vi "lapdata.vi"(6 "Reset":bool, 7 "Laptrigger":bool, 8 "InverterTemps":dbl[](array[numeric]), 9 "MotorTemps":dbl[](array[numeric]), 10 "Current":dbl, 11 "SoC":i32) -> (0 "Inverter Temp":cluster{i32[], dbl[]}[](graph), 1 "Motor Temp":cluster{i32[], dbl[]}[](graph), 3 "Lap                    Laptime                        SoC                 Current Avg |                             Motor Temperatures                          |                               Inverter Temperatures":T1(array[cluster]) {"Laptime" format="%<%M:%S%2u>T"})   [LabVIEW 2017]
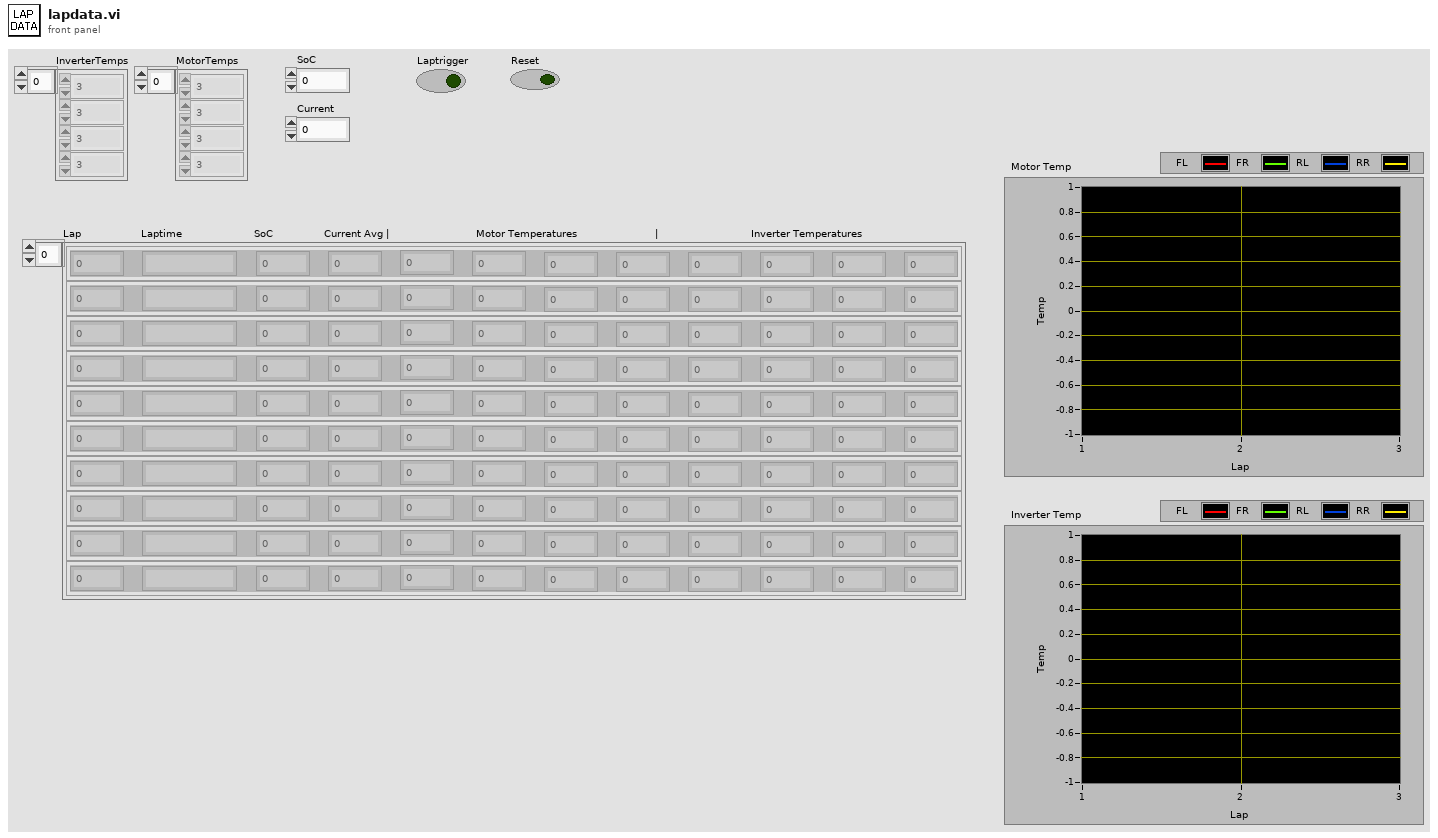
[diagram p1: front panel]
types:
  T1 = cluster{"SoC":i32, "MotorTemp_FL":dbl, "MotorTemp_FR":dbl, "MotorTemp_RL":dbl, "MotorTemp_RR":dbl, "InverterTemp_FL":dbl, "InverterTemp_FR":dbl, "InverterTemp_RL":dbl, "InverterTemp_RR":dbl, "Laptime":timestamp, "Lap":i32, "Curr Abs Avg":dbl}[]
  T2 = cluster{"SoC":i32, "MotorTemp_FL":dbl, "MotorTemp_FR":dbl, "MotorTemp_RL":dbl, "MotorTemp_RR":dbl, "InverterTemp_FL":dbl, "InverterTemp_FR":dbl, "InverterTemp_RL":dbl, "InverterTemp_RR":dbl, "Laptime":timestamp, "Lap":i32, "Current Abs Avg":dbl}[]
  T3 = cluster{"SoC":i32, "MotorTemp_FL":dbl, "MotorTemp_FR":dbl, "MotorTemp_RL":dbl, "MotorTemp_RR":dbl, "InverterTemp_FL":dbl, "InverterTemp_FR":dbl, "InverterTemp_RL":dbl, "InverterTemp_RR":dbl, "Laptime":timestamp, "Lap":i32, "Current Abs Avg":dbl}
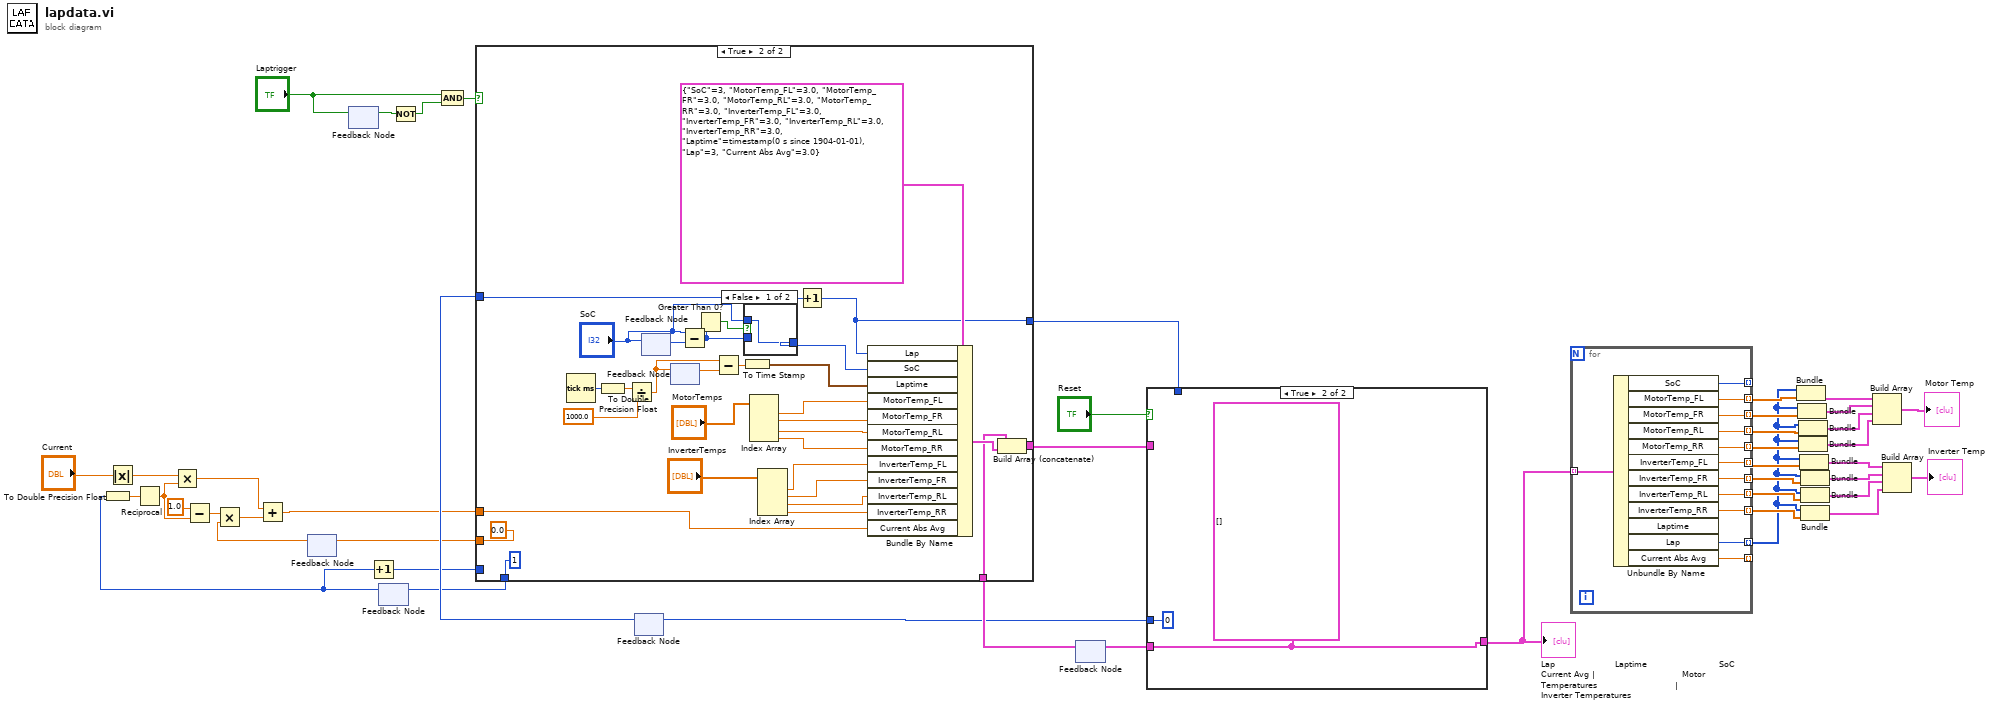
[diagram p0: block diagram]
diagram:
  n1 = Absolute Value(x="Current") -> (abs(x)=w26:dbl)
  n2 = feedback #1() -> (w30:dbl)  [unwired: 1 in]
  n3 = feedback #2() -> (w44:bool)  [unwired: 1 in]
  n4 = feedback-in #2("Laptrigger") -> ()
  n5 = feedback #3() -> (w33:i32)  [unwired: 1 in]
  n6 = To Double Precision Float(number=w33) -> (double precision float=w34:dbl)
  n7 = Reciprocal(x=w34) -> (1/x=w28:dbl)
  n8 = Multiply(x=w26, y=w28) -> (x*y=w32:dbl)
  n9 = Subtract(x=1.0, y=w28) -> (x-y=w29:dbl)
  n10 = Multiply(x=w29, y=w30) -> (x*y=w31:dbl)
  n11 = Add(x=w32, y=w31) -> (x+y=w22:dbl)
  n12 = Increment(x=w33) -> (x+1=w24:i32)
  n13 = Not(x=w44) -> (.not. x?=w43:bool)
  n14 = And(x="Laptrigger", y=w43) -> (x .and. y?=w41:bool)
  n15 = feedback #4() -> (w35:i32)  [unwired: 1 in]
  n16 = feedback #5() -> (w45:T2)  [unwired: 1 in]
  n17 = case shown="True" w41 {
    tunnel: w45 -> [w49 w60]
    tunnel: [w49 w79] -> w39
    tunnel: [w48 w58] -> w37
    tunnel: w35 -> [w48 w59]
    tunnel: w24 -> [w47 _]
    tunnel: [w47 1 ("Lap")] -> w23
    tunnel: w22 -> [w46 w54]
    tunnel: [w46 0.0] -> w21
    frame False {
    }
    frame True {
      n18 = Tick Count (ms)() -> (millisecond timer value=w68:u32)
      n19 = To Double Precision Float(number=w68) -> (double precision float=w67:dbl)
      n20 = Divide(x=w67, y=1000.0) -> (x/y=w64:dbl)
      n21 = feedback #6() -> (w57:i32)  [unwired: 1 in]
      n22 = feedback-in #6("SoC") -> ()
      n23 = feedback #7() -> (w65:dbl)  [unwired: 1 in]
      n24 = feedback-in #7(w64) -> ()
      n25 = Subtract(x="SoC", y=w57) -> (x-y=w52:i32)
      n26 = Greater Than 0?(x=w52) -> (x > 0?=w51:bool)
      n27 = Subtract(x=w64, y=w65) -> (x-y=w63:dbl)
      n28 = To Time Stamp(1:w63) -> (0:w62:timestamp)
      n29 = case shown="False" w51 {
        tunnel: w52 -> [_ w82]
        tunnel: [w81 w82] -> w53
        tunnel: "SoC" -> [w81 _]
        frame False {
        }
        frame True {
        }
      }
      n30 = Index Array(array="MotorTemps") -> (element #1=w77:dbl, element #2=w76:dbl, element #3=w75:dbl, element #4=w74:dbl)  [unwired: 4 in]
      n31 = Index Array(array="InverterTemps") -> (element #1=w72:dbl, element #2=w71:dbl, element #3=w70:dbl, element #4=w69:dbl)  [unwired: 4 in]
      n32 = Increment(x=w59) -> (x+1=w58:i32)
      n33 = Bundle By Name(cluster=T3 {"SoC"=3, "MotorTemp_FL"=3.0, "MotorTemp_FR"=3.0, "MotorTemp_RL"=3.0, "MotorTemp_RR"=3.0, "InverterTemp_FL"=3.0, "InverterTemp_FR"=3.0, "InverterTemp_RL"=3.0, "InverterTemp_RR"=3.0, "Laptime"=timestamp(0 s since 1904-01-01), "Lap"=3, "Current Abs Avg"=3.0}, "Lap"=w58, "SoC"=w53, "Laptime"=w62, "MotorTemp_FL"=w77, "MotorTemp_FR"=w76, "MotorTemp_RL"=w75, "MotorTemp_RR"=w74, "InverterTemp_FL"=w72, "InverterTemp_FR"=w71, "InverterTemp_RL"=w70, "InverterTemp_RR"=w69, "Current Abs Avg"=w54) -> (w61:T3)
      n34 = Build Array (concatenate)(w60, w61) -> (w79:T2)
    }
  }
  n35 = feedback-in #1(w21) -> ()
  n36 = feedback-in #3(w23) -> ()
  n37 = case shown="True" "Reset" {
    tunnel: [w84 w85] -> w38
    tunnel: w39 -> [w84 _]
    tunnel: [w84 w85] -> w20
    tunnel: w37 -> [w83 _]
    tunnel: [w83 0 ("Lap")] -> w36
    frame False {
    }
    frame True {
      w85 = T2 []
    }
  }
  "Lap                    Laptime                        SoC                 Current Avg |                             Motor Temperatures                          |                               Inverter Temperatures" <- w20
  n38 = feedback-in #4(w36) -> ()
  n39 = feedback-in #5(w38) -> ()
  n40 = for {
    tunnel: w20 -> [w98] mode=indexing
    tunnel: [w97] -> _ mode=indexing
    tunnel: [w96] -> w19 mode=indexing
    tunnel: [w95] -> w16 mode=indexing
    tunnel: [w94] -> w15 mode=indexing
    tunnel: [w93] -> w14 mode=indexing
    tunnel: [w92] -> w10 mode=indexing
    tunnel: [w91] -> w9 mode=indexing
    tunnel: [w90] -> w8 mode=indexing
    tunnel: [w89] -> w7 mode=indexing
    tunnel: [w88] -> _ mode=indexing
    tunnel: [w87] -> w1 mode=indexing
    n41 = Unbundle By Name(w98) -> ("SoC"=w97:i32, "MotorTemp_FL"=w96:dbl, "MotorTemp_FR"=w95:dbl, "MotorTemp_RL"=w94:dbl, "MotorTemp_RR"=w93:dbl, "InverterTemp_FL"=w92:dbl, "InverterTemp_FR"=w91:dbl, "InverterTemp_RL"=w90:dbl, "InverterTemp_RR"=w89:dbl, "Lap"=w87:i32, "Current Abs Avg"=w88:dbl)  [unwired: 1 out]
  }
  n42 = Bundle(w1, w19) -> (w18:cluster{i32[], dbl[]})  [unwired: 1 in]
  n43 = Bundle(w1, w16) -> (w13:cluster{i32[], dbl[]})  [unwired: 1 in]
  n44 = Bundle(w1, w15) -> (w12:cluster{i32[], dbl[]})  [unwired: 1 in]
  n45 = Bundle(w1, w14) -> (w11:cluster{i32[], dbl[]})  [unwired: 1 in]
  n46 = Bundle(w1, w10) -> (w5:cluster{i32[], dbl[]})  [unwired: 1 in]
  n47 = Bundle(w1, w9) -> (w4:cluster{i32[], dbl[]})  [unwired: 1 in]
  n48 = Bundle(w1, w8) -> (w3:cluster{i32[], dbl[]})  [unwired: 1 in]
  n49 = Bundle(w1, w7) -> (w2:cluster{i32[], dbl[]})  [unwired: 1 in]
  n50 = Build Array(w18, w13, w12, w11) -> (→"Motor Temp":cluster{i32[], dbl[]}[])
  n51 = Build Array(w5, w4, w3, w2) -> (→"Inverter Temp":cluster{i32[], dbl[]}[])
